vi "PH_Beckhoff.set GUI Refs.vi"(0 "i ref in":refnum<vi>, 1 "Class":string, 2 "GUI Refs":T1, 5 "error in":errorcluster) -> (14 "i ref out":refnum<vi>, 19 "error out":errorcluster)   [LabVIEW 2014, in "PH_Beckhoff.lvlib"]
uses:
  PH_Beckhoff.lvlib
  PH_Beckhoff.GUI Refs.ctl
  PH_Beckhoff.Values.ctl
  PH_Beckhoff.Sonderklemmen Inputs.ctl
  PH_Beckhoff.Analog Inputs.ctl
  PH_Beckhoff.Scaling Type.ctl
  PH_Beckhoff.Analog Outputs.ctl
  PH_Beckhoff.Digital Inputs.ctl
  PH_Beckhoff.Digital Outputs.ctl
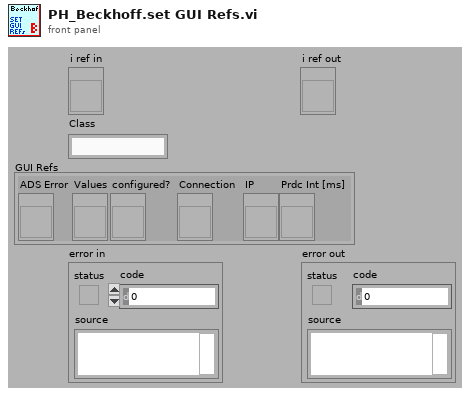
[diagram p1: front panel]
types:
  T1 = typedef "PH_Beckhoff.lvlib/PH_Beckhoff.GUI Refs.ctl" = cluster{"ADS Error":refnum<vi>, "Values":refnum<vi>, "configured?":refnum<vi>, "Connection":refnum<vi>, "IP":refnum<vi>, "Prdc Int [ms]":refnum<vi>}
  T2 = typedef "PH_Beckhoff.lvlib/PH_Beckhoff.i attribute.ctl" = cluster{"GUI Refs":T1, "operation?":bool, "Default Prdc Interval":i32, "Connection":T3, "AMS Net ID":T4, "Klemmencluster: # of":T5, "Values":T6, "IP":string, "Description":string, "configured?":bool, "Change Manager":cluster{"Detemination wanted?":bool, "Values changed at":cluster{"Sonderklemmen Inputs":i32[], "Analog Inputs":i32[], "Analog Outputs":i32[], "Digital Inputs":i32[], "Digital Outputs":i32[]}}, "Difference to handle an analog input as change":u32}
  T3 = typedef "PH_Beckhoff.lvlib/PH_Beckhoff.Connectivity.ctl" = cluster{"DLL?":bool, "Port?":bool, "Client?":bool, "Ping?":bool, "unsuccessful Pings":u32}
  T4 = typedef "Beckhoff - Driver np.lvlib/Beckhoff Access.ctl" = cluster{"DLL path":path, "AMS Net ID":cluster{"1st # of IP":u8, "2nd # of IP":u8, "3rd # of IP":u8, "4th # of IP":u8, "In Port":u8, "Out Port":u8}}
  T5 = typedef "Beckhoff - Driver np.lvlib/Klemmendeclarer.ctl" = cluster{"Offset due to Sonderklemms":u32, "analog Inputs":u32, "analog Outputs":u32, "digital Input Bits":u32, "digital Output Bits":u32}
  T6 = typedef "PH_Beckhoff.lvlib/PH_Beckhoff.Values.ctl" = cluster{"Sonderklemmen Inputs":T7, "Analog Inputs":T8, "Analog Outputs":T10, "Digital Inputs":T11, "Digital Outputs":T12}
  T7 = typedef "PH_Beckhoff.lvlib/PH_Beckhoff.Sonderklemmen Inputs.ctl" = cluster{"Total Length":u32, "Name":string, "Value":u64, "Quality":bool, "Service ID":i32, "Offset":u32, "Length":u32}[]
  T8 = typedef "PH_Beckhoff.lvlib/PH_Beckhoff.Analog Inputs.ctl" = cluster{"Name":string, "Value":u32, "Quality":bool, "Service ID":i32, "Sca Type":T9}[]
  T9 = typedef "PH_Beckhoff.lvlib/PH_Beckhoff.Scaling Type.ctl" = enum16{"none", "0 ... 15 Bit -> 0 ... 5", "0 ... 15 Bit -> 0 ... 10", "0 ... 15 Bit -> 0 ... 25", "0 ... 15 Bit -> 4 ... 20", "0 ... 15 Bit -> 0 ... 1", "0 ... 15 Bit -> 0 ... 20000", "0 ... 15 Bit -> 0 ... 24000"}
  T10 = typedef "PH_Beckhoff.lvlib/PH_Beckhoff.Analog Outputs.ctl" = cluster{"Name":string, "Value":u32, "Quality":bool, "Wanted Value":u32, "Service ID":i32, "Sca Type":T9}[]
  T11 = typedef "PH_Beckhoff.lvlib/PH_Beckhoff.Digital Inputs.ctl" = cluster{"Name":string, "Value":bool, "Quality":bool, "Service ID":i32, "inverted?":bool}[]
  T12 = typedef "PH_Beckhoff.lvlib/PH_Beckhoff.Digital Outputs.ctl" = cluster{"Name":string, "Value":bool, "Quality":bool, "Wanted Value":bool, "Service ID":i32, "inverted?":bool}[]
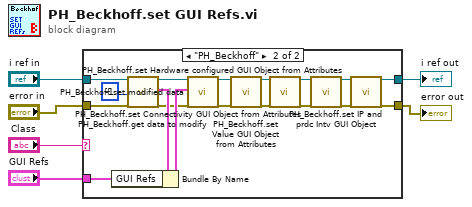
[diagram p0: block diagram]
diagram:
  n1 = case shown="\"PH_Beckhoff\"" "Class" {
    tunnel: "GUI Refs" -> [_ w26]
    tunnel: "error in" -> [w7 w23]
    tunnel: "i ref in" -> [w8 w22]
    tunnel: [w7 w9] -> w3
    tunnel: [w8 w11] -> w2
    frame Default {
    }
    frame "PH_Beckhoff" {
      n2 = call "PH_Beckhoff.get data to modify.vi"("i ref in"=w22, "ms timeout (10000)"=-1, "error in (no error)"=w23) -> ("i ref out"=w19:refnum<vi>, "i attribute"=w24:T2, "error out"=w20:errorcluster)  [unwired: 13 in, 1 out]
      n3 = Bundle By Name(cluster=w24, "GUI Refs"=w26) -> (w25:T2)
      n4 = call "PH_Beckhoff.set modified data.vi"("i ref in"=w19, "i attribute"=w25, "error in (no error)"=w20) -> ("i ref out"=w13:refnum<vi>, "error out"=w14:errorcluster)  [unwired: 15 in]
      n5 = call "PH_Beckhoff.set Value GUI Object from Attributes.vi"("i ref in"=w13, "error in"=w14) -> ("i ref out"=w18:refnum<vi>, "error out"=w17:errorcluster)  [unwired: 16 in]
      n6 = call "PH_Beckhoff.set Connectivity GUI Object from Attributes.vi"("i ref in"=w18, "error in"=w17) -> ("i ref out"=w15:refnum<vi>, "error out"=w16:errorcluster)  [unwired: 16 in]
      n7 = call "PH_Beckhoff.set Hardware configured GUI Object from Attributes.vi"("i ref in"=w15, "error in"=w16) -> ("i ref out"=w12:refnum<vi>, "error out"=w10:errorcluster)  [unwired: 16 in]
      n8 = call "PH_Beckhoff.set IP and prdc Intv GUI Object.vi"("VI in"=w12, "error in (no error)"=w10) -> ("VI out"=w11:refnum<vi>, "error out"=w9:errorcluster)  [unwired: 16 in]
    }
  }
  "error out" <- w3
  "i ref out" <- w2
